vi "Strafe Correction Voltage.vi"() -> ()   [LabVIEW 2018]
panel:
  out "Strafe Correction Voltage":dbl
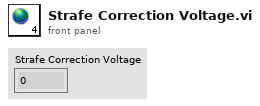
[diagram p1: front panel]
diagram:
